vi "Init_DM_V2.vi"(7 "BM Flat":bool, 8 "BM Flat File":string, 9 "Mirror Modes File":string, 10 "DM Mapping File":string, 11 "Base File Path":path) -> (3 "reference out":refnum<k7>)   [LabVIEW 2014]
uses:
  Controls/Standard Action.ctl
  <vilib>/Utility/file.llb/Read From Spreadsheet File (DBL).vi
  <vilib>/Utility/file.llb/Read From Spreadsheet File (string).vi
panel:
  out "IDs":i32[](array[numeric])
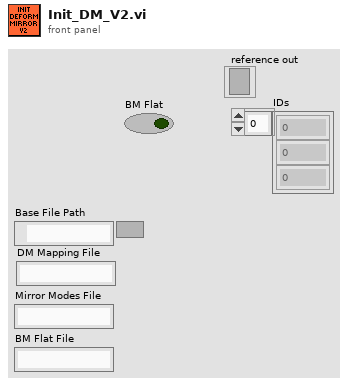
[diagram p1: front panel]
types:
  T1 = typedef "Standard Action.ctl" = enum16{"Read", "Write"}
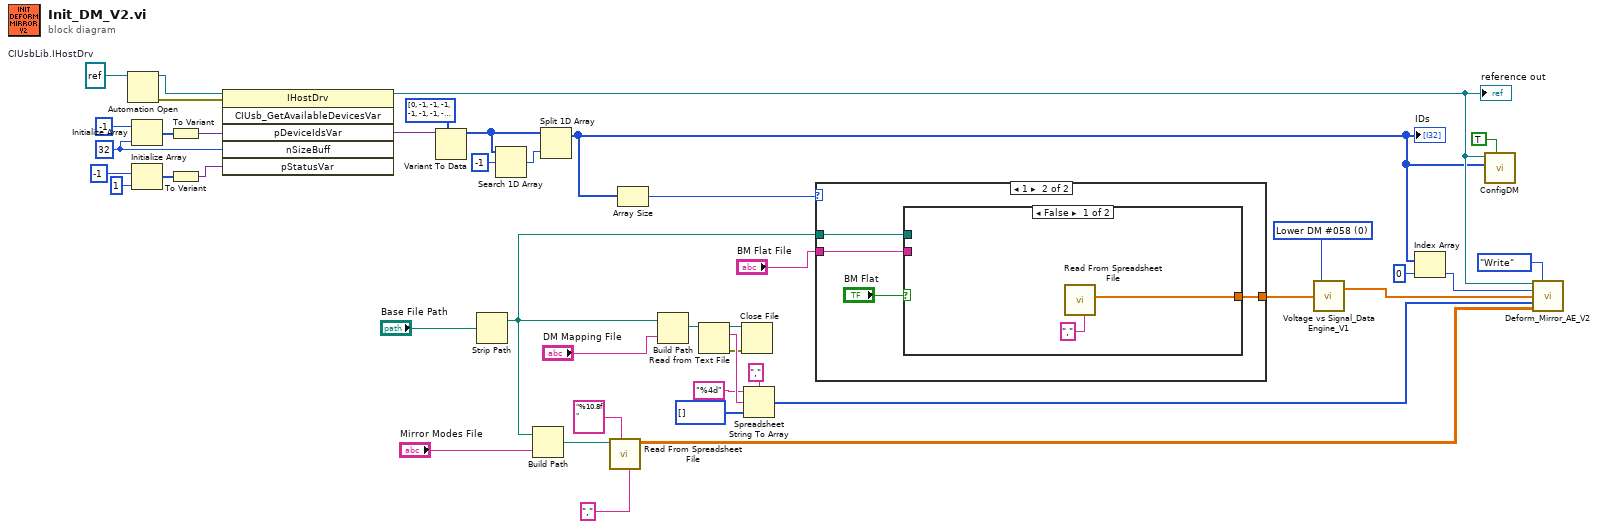
[diagram p0: block diagram]
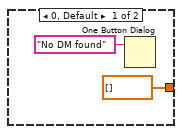
[diagram p2: hidden frame]
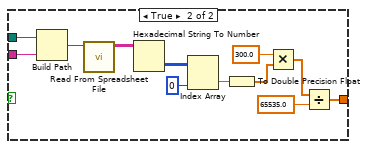
[diagram p3: hidden frame]
diagram:
  w1 = u16 0 items=["Lower DM #058", "Upper DM #029"] ("DM #")
  w38 = 32 ("dimension size")
  w29 = refnum<k7> refnum  # CIUsbLib.IHostDrv
  n1 = Automation Open(Automation Refnum=w29) -> (Automation Refnum=w34:refnum<k7>, error out=w35:errorcluster)  [unwired: 1 in, 2 out]
  n2 = Initialize Array(-1 ("element"), w38) -> (w31:i32[])
  n3 = Initialize Array(-1 ("element"), 1 ("dimension size")) -> (w30:i32[])
  n4 = To Variant(anything=w31) -> (Variant=w32:variant)
  n5 = To Variant(anything=w30) -> (Variant=w37:variant)
  n6 = invoke class="IHostDrv" method="CIUsb_GetAvailableDevicesVar"(reference=w34, error in=w35, "pDeviceIdsVar"=w32, "nSizeBuff"=w38, "pStatusVar"=w37) -> (reference out=w14:refnum<k7>, "pDeviceIdsVar"=w43:variant)  [unwired: 1 in, 4 out]
  "reference out" <- w14
  n7 = Variant To Data(type=i32[] [0, -1, -1, -1, -1, -1, -1, -1, -1, -1, -1, -1, -1, -1, -1, -1, -1, -1, -1, -1, -1, -1, -1, -1, -1, -1, -1, -1, -1, -1, -1, -1] ("pDeviceIDs"), Variant=w43) -> (data=w41:i32[])  [unwired: 1 in, 1 out]
  n8 = Strip Path(path="Base File Path") -> (stripped path=w19:path)  [unwired: 1 out]
  n9 = Search 1D Array(1D array=w41, element=-1) -> (index of element=w40:i32)  [unwired: 1 in]
  n10 = Build Path(base path=w19, name or relative path="Mirror Modes File") -> (appended path=w20:path)
  n11 = Split 1D Array(array=w41, index=w40) -> (first subarray=w13:i32[])  [unwired: 1 out]
  "IDs" <- w13
  n12 = call-poly <vilib>:"Read From Spreadsheet File.vi"("delimiter (\\t)"="," ("delimiter (\\t)"), "format (%.3f)"="%10.8f", "file path (dialog if empty)"=w20) -> ("all rows"=w5:dbl[][])  [unwired: 2 in, 6 out]
  n13 = Array Size(array=w13) -> (size(s)=w17:i32)
  n14 = Build Path(base path=w19, name or relative path="DM Mapping File") -> (appended path=w22:path)
  n15 = Read from Text File(file (use dialog)=w22) -> (refnum out=w24:refnum<file>, text=w28:string, error out=w23:errorcluster)  [unwired: 1 in, 3 out]
  n16 = Close File(refnum=w24, error in=w23) -> ()  [unwired: 2 out]
  n17 = Spreadsheet String To Array(delimiter (Tab)=",", format string="%4d", spreadsheet string=w28, array type (2D Dbl)=i32[] []) -> (array=w16:i32[])
  n18 = case shown="1" w17 {
    tunnel: w19 -> [_ w49]
    tunnel: "BM Flat File" -> [_ w48]
    tunnel: [dbl[] [] w47] -> w3
    frame 0, Default {
      n19 = One Button Dialog(message="No DM found") -> ()  [unwired: 1 in, 1 out]
    }
    frame 1 {
      n20 = case shown="False" "BM Flat" {
        tunnel: w49 -> [_ w63]
        tunnel: w48 -> [_ w62]
        tunnel: [w50 w53] -> w47
        frame False {
          n21 = call-poly <vilib>:"Read From Spreadsheet File.vi"("delimiter (\\t)"="," ("delimiter (\\t)")) -> ("first row"=w50:dbl[])  [unwired: 6 in, 4 out]
        }
        frame True {
          n22 = Build Path(base path=w63, name or relative path=w62) -> (appended path=w61:path)
          n23 = call-poly <vilib>:"Read From Spreadsheet File.vi"("file path (dialog if empty)"=w61) -> ("all rows"=w60:string[][])  [unwired: 3 in, 7 out]
          n24 = Hexadecimal String To Number(string=w60) -> (number=w59:u32[][])  [unwired: 2 in, 1 out]
          n25 = Index Array(array=w59, index (col)=0 ("disabled index (col)")) -> (element=w57:u32[])  [unwired: 1 in]
          n26 = To Double Precision Float(number=w57) -> (double precision float=w52:dbl[])
          n27 = Multiply(x=300.0 ("y"), y=w52) -> (x*y=w56:dbl[])
          n28 = Divide(x=w56, y=65535.0) -> (x/y=w53:dbl[])
        }
      }
    }
  }
  n29 = call "Voltage vs Signal_Data Engine_V1.vi"("Voltage in (0~Max. Vol.)"=w3, "DM #"=w1) -> ("Control Signal Out (-1~1)"=w2:dbl[])  [unwired: 1 in, 1 out]
  n30 = Index Array(array=w13, index=0) -> (element=w12:i32)
  n31 = call "ConfigDM.vi"("High Voltage"=TRUE, "Dev IDs"=w13, "Automation Refnum in"=w14) -> ()  [unwired: 7 in, 2 out]
  n32 = call "Deform_Mirror_AE_V2.vi"("Refnum In"=w14, "Action"=Standard_Action."Write", "IDs In"=w12, "Flat Files In"=w2, "Multi Map Data In"=w16, "Mode Matrix"=w5) -> ()  [unwired: 5 in, 5 out]
